vi "Next Item Object Fmily.vi"(11 "Bytes IN":u8[](array[numeric]) format="%x") -> (2 "Object Family":T2)   [LabVIEW 2020]
uses:
  MessagePack.lvclass/MessagePack.ctl
  Object Family.ctl
  MessagePack.lvclass
  MsgPack Object Types.ctl
panel:
  in  "Type":T1=enum."NEGINT"
  out "Bytes out":u8[](array[numeric]) format="%x"
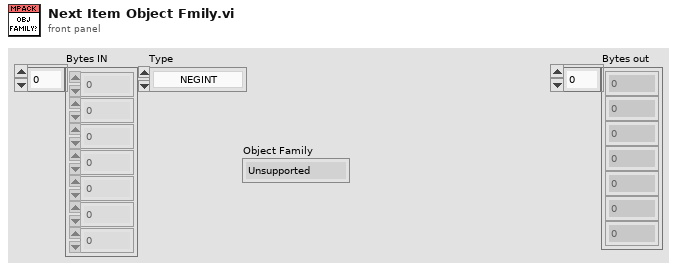
[diagram p1: front panel]
types:
  T1 = typedef "MessagePack.lvlib/MessagePack.lvclass/MsgPack Object Types.ctl" = enum16{"UNSUPPORTED", "POSINT", "NEGINT", "FIXMAP", "FIXARRAY", "FIXSTR", "NIL", "FALSE", "TRUE", "BIN8", "BIN16", "BIN32", "EXT8", "EXT16", "EXT32", "FLOAT32", "FLOAT64", "UINT8", "UINT16", "UINT32", "UINT64", "INT8", "INT16", "INT32", "INT64", "FIXEXT1", "FIXEXT2", "FIXEXT4", "FIXEXT8", "FIXEXT16", "STR8", "STR16", "STR32", "ARRAY16", "ARRAY32", "MAP16", "MAP32"}
  T2 = typedef "MessagePack.lvlib/MessagePack.lvclass/Object Family.ctl" = enum16{"Unsupported", "Nil", "Numeric", "Array", "Map", "String", "Binary", "Boolean", "Ext"}
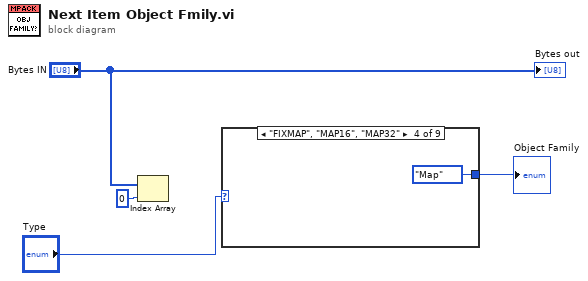
[diagram p0: block diagram]
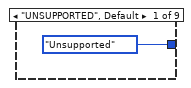
[diagram p2: hidden frame]
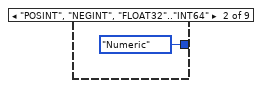
[diagram p3: hidden frame]
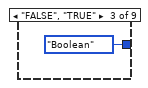
[diagram p4: hidden frame]
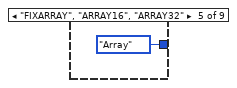
[diagram p5: hidden frame]
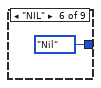
[diagram p6: hidden frame]
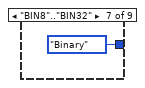
[diagram p7: hidden frame]
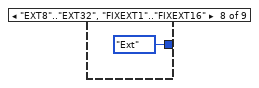
[diagram p8: hidden frame]
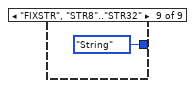
[diagram p9: hidden frame]
diagram:
  n1 = Index Array(array="Bytes IN", index=0) -> ()  [unwired: 1 out]
  n2 = case shown="\"FIXMAP\", \"MAP16\", \"MAP32\"" "Type" {
    tunnel: [Object_Family."Unsupported" ("Object Family") Object_Family."Numeric" ("Object Family") Object_Family."Boolean" ("Object Family") Object_Family."Map" ("Object Family") Object_Family."Array" ("Object Family") Object_Family."Nil" ("Object Family") Object_Family."Binary" ("Object Family") Object_Family."Ext" ("Object Family") Object_Family."String" ("Object Family")] -> w2
    frame "UNSUPPORTED", Default {
    }
    frame "POSINT", "NEGINT", "FLOAT32".."INT64" {
    }
    frame "FALSE", "TRUE" {
    }
    frame "FIXMAP", "MAP16", "MAP32" {
    }
    frame "FIXARRAY", "ARRAY16", "ARRAY32" {
    }
    frame "NIL" {
    }
    frame "BIN8".."BIN32" {
    }
    frame "EXT8".."EXT32", "FIXEXT1".."FIXEXT16" {
    }
    frame "FIXSTR", "STR8".."STR32" {
    }
  }
  "Object Family" <- w2
  "Bytes out" <- "Bytes IN"
